vi "ROI entry screen-Detect Variable Length.vi"(8 "error in (no error)":errorcluster, 11 "XYZ_Coordinates":T1[](array[typedef]) {"Apparent Frame Size" format="%#_6f"; "Original FOV (um)" format="%#_6f"; "Pixels per miniscan" format="%#_6f"; "Dwell Time per pixel" format="%#_6f"; "Resolution" format="%#_6f"; "ROI group ID" format="%#_6f"; "Laser Power (%)" format="%#_6f"; "Zoom" format="%#_6f"; "Frame Size" format="%#_6f"; "Number of lines" format="%#_6f"; "Composite ID" format="%#_6f"; "Angle (deg)" format="%#_6f"; "ROI Time (ns)" format="%#_6f"; "ROI ID" format="%#_6f"; "Pixels in ROI" format="%#_6f"; "ROI index" format="%#_6f"; "Z stop" format="%#_6f"; "Y stop" format="%#_6f"; "X stop" format="%#_6f"; "Z start" format="%#_6f"; "X start" format="%#_6f"; "Y start" format="%#_6f"}) -> (0 "error out":errorcluster, 2 "VR ?":bool, 3 "VL ?":bool)   [LabVIEW 2020]
uses:
  Visualisation/Functional Imaging Viewer/Typedefs/ROI parameters data type.ctl
  Typedefs/ROI ID Enum.ctl
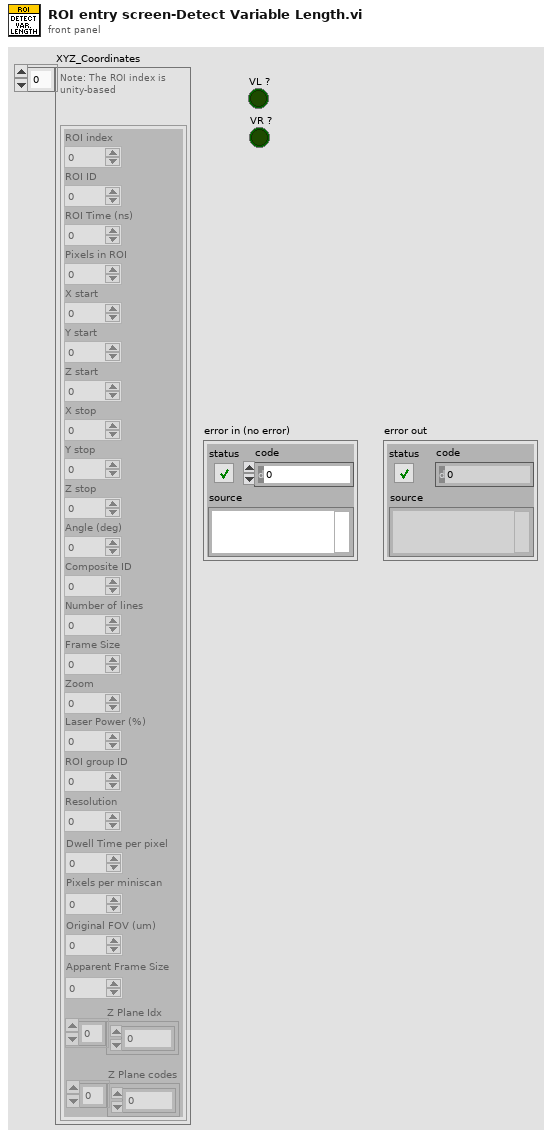
[diagram p1: front panel]
types:
  T1 = typedef "ROI parameters data type.ctl" = cluster{"ROI index":dbl, "ROI ID":dbl, "ROI Time (ns)":dbl, "Pixels in ROI":dbl, "X start":dbl, "Y start":dbl, "Z start":dbl, "X stop":dbl, "Y stop":dbl, "Z stop":dbl, "Angle (deg)":dbl, "Composite ID":dbl, "Number of lines":dbl, "Frame Size":dbl, "Zoom":dbl, "Laser Power (%)":dbl, "ROI group ID":dbl, "Resolution":dbl, "Dwell Time per pixel":dbl, "Pixels per miniscan":dbl, "Original FOV (um)":dbl, "Apparent Frame Size":dbl, "Z Plane Idx":i32[], "Z Plane codes":i32[]}
  T2 = typedef "ROI ID Enum.ctl" = enum16{"Point", "MiniScan", "Comp. MiniScan", "Rectangle", "Comp. volume", "Arb. plane point", "None"}
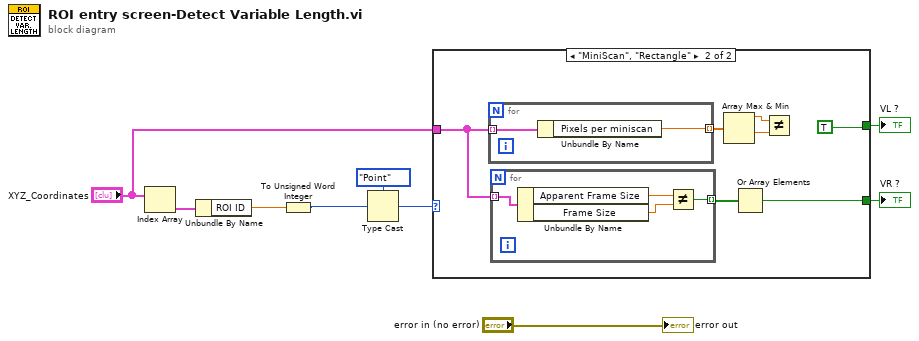
[diagram p0: block diagram]
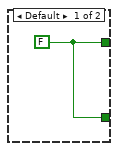
[diagram p2: hidden frame]
diagram:
  n1 = Index Array(array="XYZ_Coordinates") -> (element=w8:T1)  [unwired: 1 in]
  n2 = Unbundle By Name(w8) -> ("ROI ID"=w7:dbl)
  n3 = To Unsigned Word Integer(number=w7) -> (unsigned 16bit integer=w1:u16)
  n4 = Type Cast(type=ROI_ID_Enum."Point" ("ROI ID Enum"), x=w1) -> (*(type *) &x=w6:T2)
  n5 = case shown="\"MiniScan\", \"Rectangle\"" w6 {
    tunnel: "XYZ_Coordinates" -> [_ w14]
    tunnel: [w10 TRUE] -> w3
    tunnel: [w10 w12] -> w2
    frame Default {
      w10 = FALSE
    }
    frame "MiniScan", "Rectangle" {
      n6 = for {
        tunnel: w14 -> [w23] mode=indexing
        tunnel: [w22] -> w17 mode=indexing
        n7 = Unbundle By Name(w23) -> ("Pixels per miniscan"=w22:dbl)
      }
      n8 = for {
        tunnel: w14 -> [w21] mode=indexing
        tunnel: [w19] -> w13 mode=indexing
        n9 = Unbundle By Name(w21) -> ("Apparent Frame Size"=w20:dbl, "Frame Size"=w18:dbl)
        n10 = Not Equal?(x=w20, y=w18) -> (x != y?=w19:bool)
      }
      n11 = Array Max & Min(array=w17) -> (max value=w16:dbl, min value=w15:dbl)  [unwired: 2 out]
      n12 = Or Array Elements(Boolean array=w13) -> (logical OR=w12:bool)
      n13 = Not Equal?(x=w16, y=w15) -> ()  [unwired: 1 out]
    }
  }
  "VL ?" <- w3
  "VR ?" <- w2
  "error out" <- "error in (no error)"
